vi "Glyph Index.vi"(8 "error in (no error)":errorcluster, 11 "Valve Item in":refnum<class "Valve Item.lvclass">) -> (0 "error out":errorcluster, 2 "Glyph Index":i32, 3 "Valve Item out":refnum<class "Valve Item.lvclass">)   [LabVIEW 2020, in "BetterDragAndDropDemo.lvlib" / "Valve Item.lvclass"]
uses:
  Valve Item.lvclass
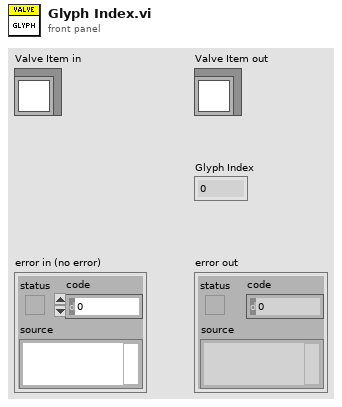
[diagram p1: front panel]
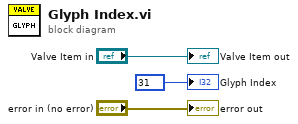
[diagram p0: block diagram]
diagram:
  "error out" <- "error in (no error)"
  "Valve Item out" <- "Valve Item in"
  "Glyph Index" <- 31
